vi "Pre-Build_Test_Stub.vi"(6 "Top Level/Always Included VIs":path[](array[path]), 7 "Main Destination Path":path, 9 "Target Name":string, 10 "Build Specification Name":string, 11 "Project Path":path) -> (0 "error out":errorcluster)   [LabVIEW 2020]
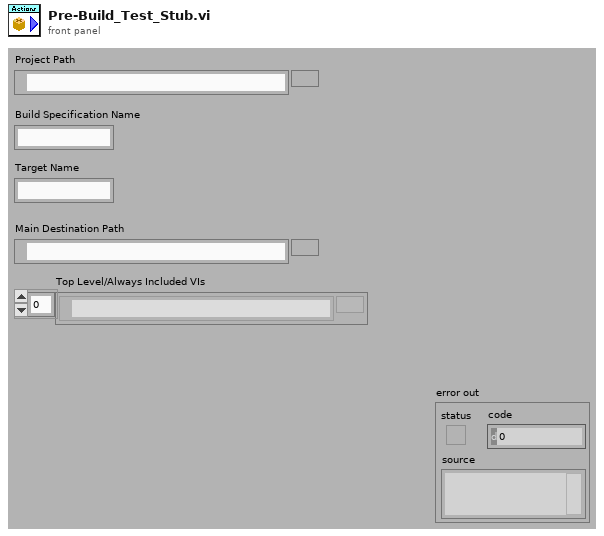
[diagram p1: front panel]
types:
  T1 = enum16{"open", "replace", "create", "open or create", "replace or create", "replace or create with confirmation"}
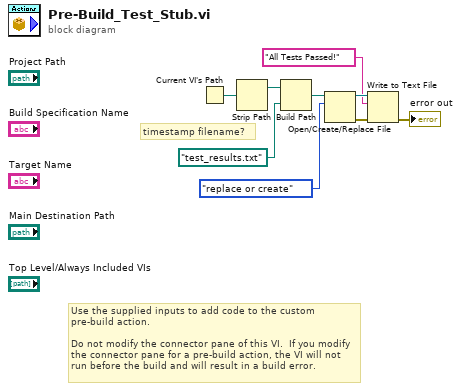
[diagram p0: block diagram]
diagram:
  # "timestamp filename?"
  # "Use the supplied inputs to add code to the custom pre-build action.\n\nDo not modify the connector pane of this VI.  If you modify the connector pane for a pre-build action, the VI will not run before the build and will result in a build error."
  n1 = Current VI's Path() -> (path=w9:path)
  n2 = Strip Path(path=w9) -> (stripped path=w8:path)  [unwired: 1 out]
  n3 = Build Path(base path=w8, name or relative path=path "test_results.txt") -> (appended path=w6:path)
  n4 = Open/Create/Replace File(file path (use dialog)=w6, operation (0:open)=T1."replace or create") -> (refnum out=w4:refnum<file>, error out=w3:errorcluster)  [unwired: 4 in, 1 out]
  n5 = Write to Text File(file (use dialog)=w4, text="All Tests Passed!", error in=w3) -> (error out=→"error out":errorcluster)  [unwired: 1 in, 2 out]
